vi "reenable fp controls after flystart.vi"() -> ()   [LabVIEW 2017]
doc: "SciScan 1.2 160622"
uses:
  Custom Controls/pixel resolution enum.ctl
  GFG/GFGfpRefGet.vi
  GFG/GFG library.lvlib
panel:
  out "error out 5":errorcluster
  out "error out 4":errorcluster
  out "error out 3":errorcluster
  out "error out 2":errorcluster
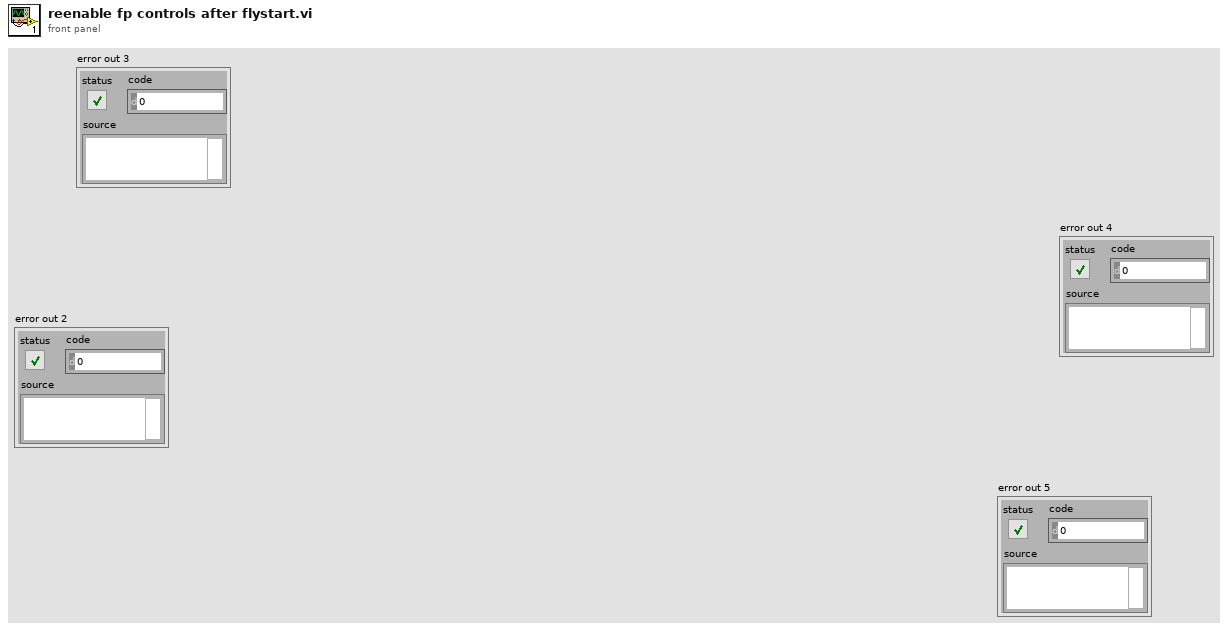
[diagram p1: front panel]
types:
  T1 = typedef "pixel resolution enum.ctl" = enum16{"128 x 128", "256 x 128", "256 x 256", "512 x  64", "512 x 128", "512 x 256", "512 x 512", "1024 x 512", "1024 x 1024", "arbitrary"}
  T2 = enum8{"Enabled", "Disabled", "Disabled and Grayed Out"}
  T3 = cluster{"WaveformChartRef":refnum<vi>, "DigitalRef":refnum<vi>, "ArrayRef":refnum<vi>, "TabControlRef":refnum<vi>, "EnumRef":refnum<vi>, "RingRef":refnum<vi>, "BooleanRef":refnum<vi>, "KnobRef":refnum<vi>, "SlideRef":refnum<vi>, "PathRef":refnum<vi>, "StringRef":refnum<vi>, "ComboBox":refnum<vi>, "WaveformGraphRef":refnum<vi>}
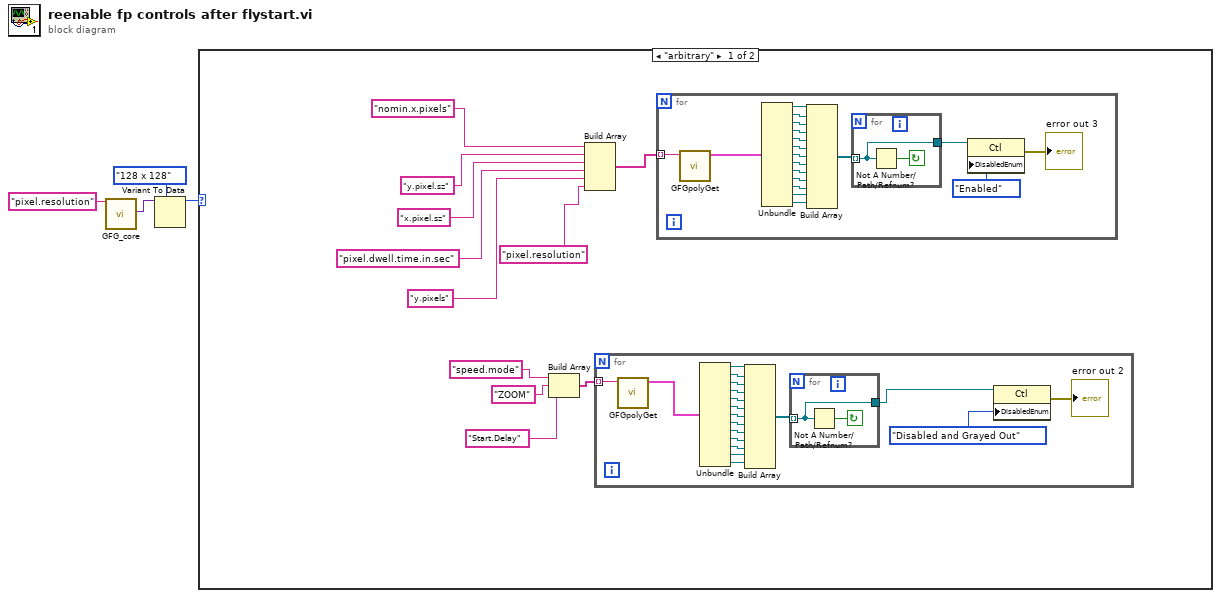
[diagram p0: block diagram]
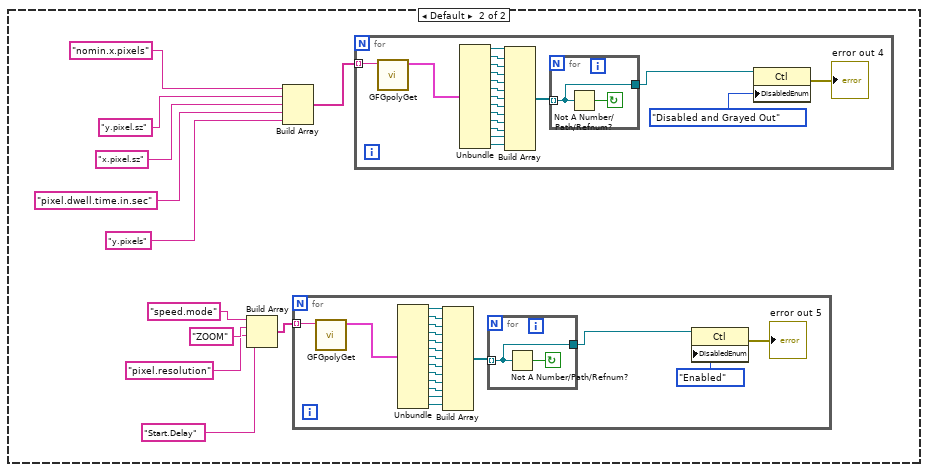
[diagram p2: hidden frame]
diagram:
  n1 = call "GFG_core.vi"("Variable Name in"="pixel.resolution") -> ("Variant Out"=w2:variant)  [unwired: 12 in, 6 out]
  n2 = Variant To Data(type=pixel_resolution_enum."128 x 128" ("pixel resolution"), Variant=w2) -> (data=w1:T1)  [unwired: 1 in, 1 out]
  n3 = case shown="\"arbitrary\"" w1 {
    frame "arbitrary" {
      n4 = Build Array("speed.mode" ("Variable Name in"), "ZOOM" ("Variable Name in"), "Start.Delay" ("Variable Name in")) -> (w8:string[])
      n5 = Build Array("nomin.x.pixels" ("Variable Name in"), "y.pixel.sz" ("Variable Name in"), "x.pixel.sz" ("Variable Name in"), "pixel.dwell.time.in.sec" ("Variable Name in"), "y.pixels" ("Variable Name in"), "pixel.resolution" ("element")) -> (w7:string[])
      n6 = for {
        tunnel: w8 -> [w41] mode=indexing
        n7 = call-poly "GFGpolyGet.vi"("Variable Name in"=w41) -> ("output cluster"=w42:T3)  [unwired: 9 in, 1 out]
        n8 = Unbundle(w42) -> ("WaveformChartRef"=w37:refnum<vi>, "DigitalRef"=w44:refnum<vi>, "ArrayRef"=w45:refnum<vi>, "TabControlRef"=w46:refnum<vi>, "EnumRef"=w47:refnum<vi>, "RingRef"=w48:refnum<vi>, "BooleanRef"=w49:refnum<vi>, "KnobRef"=w50:refnum<vi>, "SlideRef"=w51:refnum<vi>, "PathRef"=w52:refnum<vi>, "StringRef"=w53:refnum<vi>, "ComboBox"=w39:refnum<vi>, "WaveformGraphRef"=w38:refnum<vi>)
        n9 = Build Array(w37, w44, w45, w46, w47, w48, w49, w50, w51, w52, w53, w39, w38) -> (w43:refnum<vi>[])
        n10 = for {
          tunnel: w43 -> [w56] mode=indexing
          tunnel: [w56] -> w40
          stop <- w57 continue-if-true
          n11 = Not A Number/Path/Refnum?(number/path/refnum=w56) -> (NaN/Path/Refnum?=w57:bool)
        }
        n12 = property class="Ctl"(reference=w40, "DisabledEnum"=T2."Disabled and Grayed Out" ("Disabled")) -> (error out=→"error out 2":errorcluster)  [unwired: 1 in, 1 out]
      }
      n13 = for {
        tunnel: w7 -> [w20] mode=indexing
        n14 = call-poly "GFGpolyGet.vi"("Variable Name in"=w20) -> ("output cluster"=w21:T3)  [unwired: 9 in, 1 out]
        n15 = Unbundle(w21) -> ("WaveformChartRef"=w16:refnum<vi>, "DigitalRef"=w23:refnum<vi>, "ArrayRef"=w24:refnum<vi>, "TabControlRef"=w25:refnum<vi>, "EnumRef"=w26:refnum<vi>, "RingRef"=w27:refnum<vi>, "BooleanRef"=w28:refnum<vi>, "KnobRef"=w29:refnum<vi>, "SlideRef"=w30:refnum<vi>, "PathRef"=w31:refnum<vi>, "StringRef"=w32:refnum<vi>, "ComboBox"=w18:refnum<vi>, "WaveformGraphRef"=w17:refnum<vi>)
        n16 = Build Array(w16, w23, w24, w25, w26, w27, w28, w29, w30, w31, w32, w18, w17) -> (w22:refnum<vi>[])
        n17 = for {
          tunnel: w22 -> [w35] mode=indexing
          tunnel: [w35] -> w19
          stop <- w36 continue-if-true
          n18 = Not A Number/Path/Refnum?(number/path/refnum=w35) -> (NaN/Path/Refnum?=w36:bool)
        }
        n19 = property class="Ctl"(reference=w19, "DisabledEnum"=T2."Enabled" ("Disabled")) -> (error out=→"error out 3":errorcluster)  [unwired: 1 in, 1 out]
      }
    }
    frame Default {
      n20 = Build Array("speed.mode" ("Variable Name in"), "ZOOM" ("Variable Name in"), "pixel.resolution" ("element"), "Start.Delay" ("Variable Name in")) -> (w61:string[])
      n21 = Build Array("nomin.x.pixels" ("Variable Name in"), "y.pixel.sz" ("Variable Name in"), "x.pixel.sz" ("Variable Name in"), "pixel.dwell.time.in.sec" ("Variable Name in"), "y.pixels" ("Variable Name in")) -> (w60:string[])
      n22 = for {
        tunnel: w61 -> [w94] mode=indexing
        n23 = call-poly "GFGpolyGet.vi"("Variable Name in"=w94) -> ("output cluster"=w95:T3)  [unwired: 9 in, 1 out]
        n24 = Unbundle(w95) -> ("WaveformChartRef"=w90:refnum<vi>, "DigitalRef"=w97:refnum<vi>, "ArrayRef"=w98:refnum<vi>, "TabControlRef"=w99:refnum<vi>, "EnumRef"=w100:refnum<vi>, "RingRef"=w101:refnum<vi>, "BooleanRef"=w102:refnum<vi>, "KnobRef"=w103:refnum<vi>, "SlideRef"=w104:refnum<vi>, "PathRef"=w105:refnum<vi>, "StringRef"=w106:refnum<vi>, "ComboBox"=w92:refnum<vi>, "WaveformGraphRef"=w91:refnum<vi>)
        n25 = Build Array(w90, w97, w98, w99, w100, w101, w102, w103, w104, w105, w106, w92, w91) -> (w96:refnum<vi>[])
        n26 = for {
          tunnel: w96 -> [w109] mode=indexing
          tunnel: [w109] -> w93
          stop <- w110 continue-if-true
          n27 = Not A Number/Path/Refnum?(number/path/refnum=w109) -> (NaN/Path/Refnum?=w110:bool)
        }
        n28 = property class="Ctl"(reference=w93, "DisabledEnum"=T2."Enabled" ("Disabled")) -> (error out=→"error out 5":errorcluster)  [unwired: 1 in, 1 out]
      }
      n29 = for {
        tunnel: w60 -> [w73] mode=indexing
        n30 = call-poly "GFGpolyGet.vi"("Variable Name in"=w73) -> ("output cluster"=w74:T3)  [unwired: 9 in, 1 out]
        n31 = Unbundle(w74) -> ("WaveformChartRef"=w69:refnum<vi>, "DigitalRef"=w76:refnum<vi>, "ArrayRef"=w77:refnum<vi>, "TabControlRef"=w78:refnum<vi>, "EnumRef"=w79:refnum<vi>, "RingRef"=w80:refnum<vi>, "BooleanRef"=w81:refnum<vi>, "KnobRef"=w82:refnum<vi>, "SlideRef"=w83:refnum<vi>, "PathRef"=w84:refnum<vi>, "StringRef"=w85:refnum<vi>, "ComboBox"=w71:refnum<vi>, "WaveformGraphRef"=w70:refnum<vi>)
        n32 = Build Array(w69, w76, w77, w78, w79, w80, w81, w82, w83, w84, w85, w71, w70) -> (w75:refnum<vi>[])
        n33 = for {
          tunnel: w75 -> [w88] mode=indexing
          tunnel: [w88] -> w72
          stop <- w89 continue-if-true
          n34 = Not A Number/Path/Refnum?(number/path/refnum=w88) -> (NaN/Path/Refnum?=w89:bool)
        }
        n35 = property class="Ctl"(reference=w72, "DisabledEnum"=T2."Disabled and Grayed Out" ("Disabled")) -> (error out=→"error out 4":errorcluster)  [unwired: 1 in, 1 out]
      }
    }
  }
